vi "Time to Seconds.vi"(8 "Seconds":dbl=1.0 format="%#.6f", 9 "Minutes":dbl=1.0, 10 "Hours":dbl=1.0, 11 "Days":dbl=1.0) -> (3 "Time Goal (s)":dbl=1.0 format="%#.6f")   [LabVIEW 2021, in "Timer-API.lvlib" / "Timer Session.lvclass"]
doc: "Calculate seconds from days, hours, minutes and seconds. The output can be used as timer target in Timer API."
uses:
  Timer Session.lvclass
  Timer Session.lvclass/Timer Session.ctl
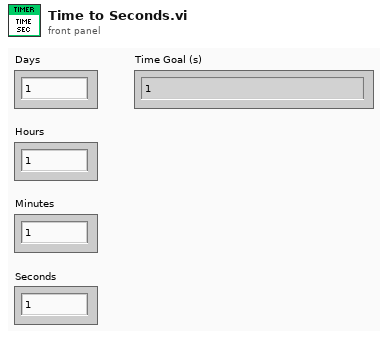
[diagram p1: front panel]
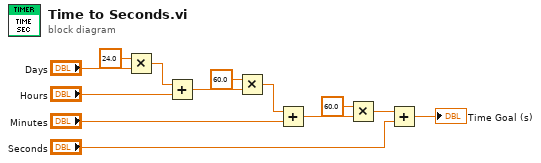
[diagram p0: block diagram]
diagram:
  n1 = Multiply(x=24.0, y="Days") -> (x*y=w11:dbl)
  n2 = Add(x=w11, y="Hours") -> (x+y=w9:dbl)
  n3 = Multiply(x=60.0, y=w9) -> (x*y=w7:dbl)
  n4 = Add(x=w7, y="Minutes") -> (x+y=w4:dbl)
  n5 = Multiply(x=60.0, y=w4) -> (x*y=w3:dbl)
  n6 = Add(x=w3, y="Seconds") -> (x+y=→"Time Goal (s)":dbl)
